vi "Add VI to class library.vi"(8 "Error In":errorcluster, 10 "New method path":path, 11 "Class Ref":refnum<vi>) -> (0 "Error Out":errorcluster)   [LabVIEW 2013, in "Scripter.lvlib"]
uses:
  Scripter.lvlib
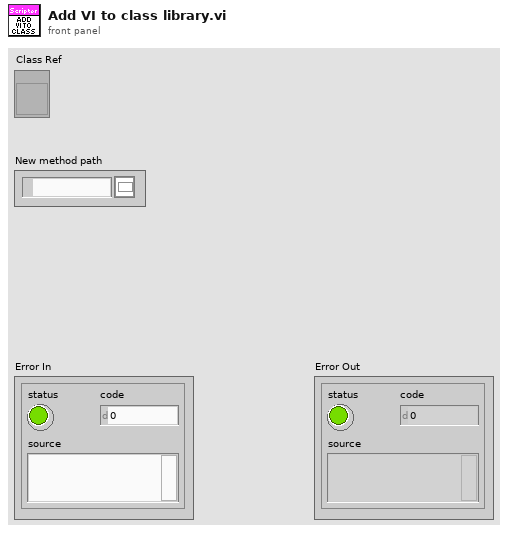
[diagram p1: front panel]
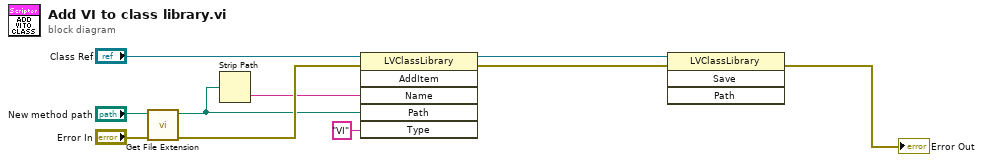
[diagram p0: block diagram]
diagram:
  n1 = call <vilib>:"Get File Extension.vi"("error in (no error)"="Error In", "file"="New method path") -> ("error out"=w6:errorcluster, "dup file"=w1:path)  [unwired: 6 in, 2 out]
  n2 = Strip Path(path=w1) -> (name=w2:string)  [unwired: 1 out]
  n3 = invoke class="LVClassLibrary" method="AddItem"(reference="Class Ref", error in=w6, "Name"=w2, "Path"=w1, "Type"="VI") -> (reference out=w5:refnum<vi>, error out=w4:errorcluster)  [unwired: 1 in, 4 out]
  n4 = invoke class="LVClassLibrary" method="Save"(reference=w5, error in=w4) -> (error out=→"Error Out":errorcluster)  [unwired: 2 in, 3 out]
